vi "practica4rio.vi"() -> ()   [LabVIEW 2017]
uses:
  <vilib>/addons/Fuzzy Logic/FL Fuzzy Controller (SIMO).vi
  <vilib>/addons/Fuzzy Logic/NI_Fuzzy_Logic_API.lvlib
panel:
  out "motor izquierdo":dbl[](graph)
  out "motor derecho":dbl[](graph)
  in  "file path 2":path
  in  "Reset":bool
  out "Distancia":dbl
  out "Angulo":dbl
  out "Motor Izquierda":dbl(slide) scale=-100.0..100.0
  out "Motor Derecha":dbl(slide) scale=-100.0..100.0
  out "Plano de trabajo":picture
  in  "stop":bool
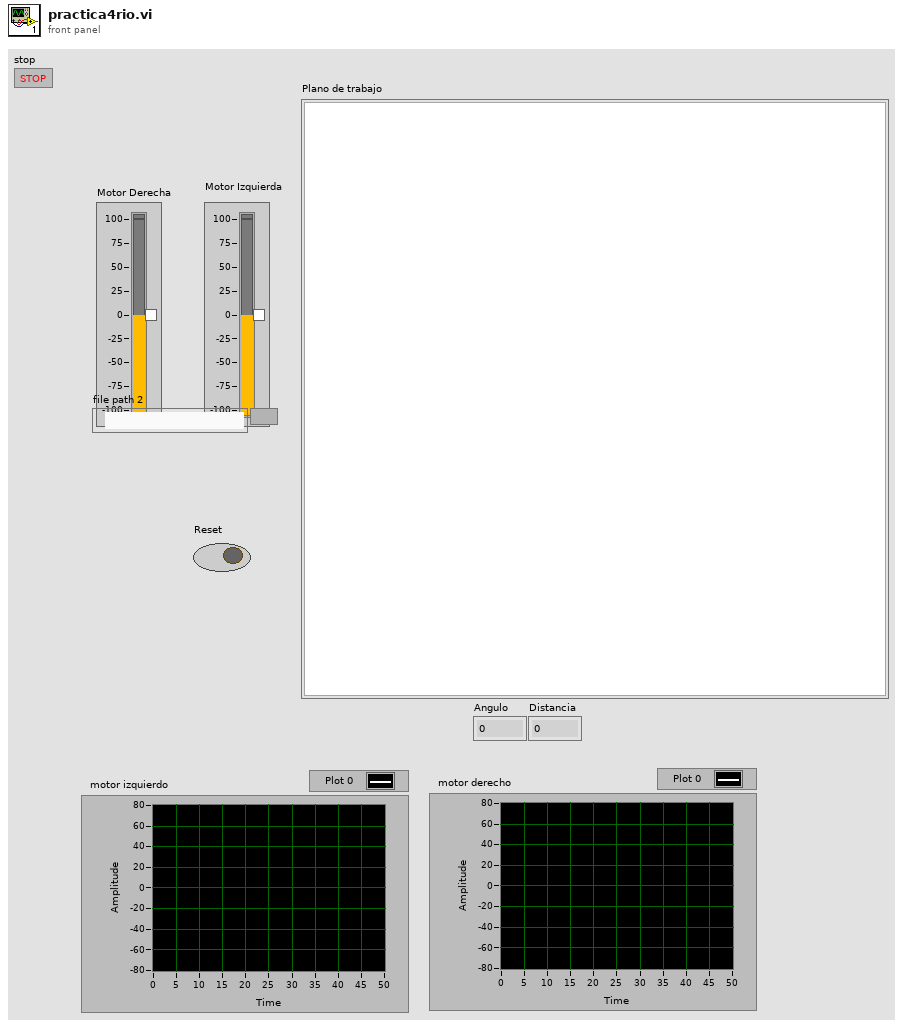
[diagram p1: front panel]
types:
  T1 = typedef "NI_Fuzzy_Logic_API.lvlib/FL System.ctl" = cluster{"input variables":T2[], "output variables":T2[], "rules":T5[], "defuzzification method":T11, "description":string, "user MF interpolating polynomials":T12[]}
  T2 = typedef "NI_Fuzzy_Logic_API.lvlib/FL Variable.ctl" = cluster{"name":string, "range":dbl[], "MFs":T3[]}
  T3 = typedef "NI_Fuzzy_Logic_API.lvlib/FL Membership Function.ctl" = cluster{"name":string, "shape":T4, "points":dbl[], "color":u32, "user-defined shape index":i32}
  T4 = typedef "NI_Fuzzy_Logic_API.lvlib/FL Membership Function Shape.ctl" = u16
  T5 = typedef "NI_Fuzzy_Logic_API.lvlib/FL Rule.ctl" = cluster{"antecedents":T6[], "antecedent connective":T8, "consequents":T9[], "consequent implication":T10, "degree of support":dbl}
  T6 = typedef "NI_Fuzzy_Logic_API.lvlib/FL Antecedent.ctl" = cluster{"Var Index":i32, "MF Index":i32, "Cond":T7}
  T7 = typedef "NI_Fuzzy_Logic_API.lvlib/FL Modifier.ctl" = u16
  T8 = typedef "NI_Fuzzy_Logic_API.lvlib/FL Antecedent Connective.ctl" = u16
  T9 = typedef "NI_Fuzzy_Logic_API.lvlib/FL Consequent.ctl" = cluster{"Var Index":i32, "MF Index":i32, "Cond":T7}
  T10 = typedef "NI_Fuzzy_Logic_API.lvlib/FL Consequent Implication.ctl" = u16
  T11 = typedef "NI_Fuzzy_Logic_API.lvlib/FL Defuzzification.ctl" = u16
  T12 = typedef "NI_Fuzzy_Logic_API.lvlib/FL Interpolating polynomials.ctl" = cluster{"X":dbl[], "Y":dbl[], "Y(x) coeff":dbl[][], "X(y) coeff":dbl[][], "Area(y) coeff":dbl[][], "coa_x(y) coeff":dbl[][]}
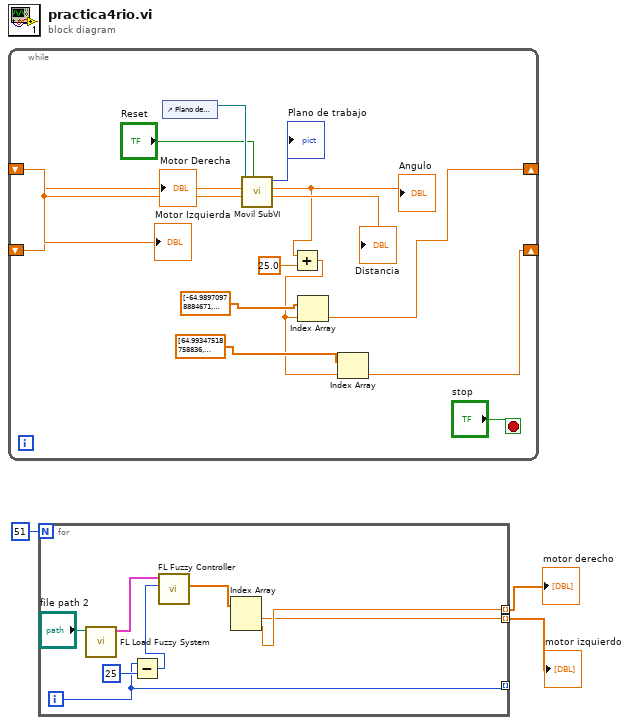
[diagram p0: block diagram]
diagram:
  n1 = while {
    shift-right: [w8] -> _
    shift-left: _ -> [w12]
    shift-right: [w7] -> _
    shift-left: _ -> [w11]
    stop <- "stop" stop-if-true
    n2 = control-ref of="Plano de trabajo"() -> (w15:refnum<vi>)
    n3 = call "Movil SubVI.vi"("Reset"="Reset", "Motor Izquierda"=w12, "Motor Derecha"=w11, "Ref Plano"=w15) -> ("Distancia"=→"Distancia":dbl, "Angulo"=w5:dbl, "Plano de trabajo"=→"Plano de trabajo":picture)  [unwired: 3 in, 2 out]
    "Angulo" <- w5
    n4 = Add(x=w5, y=25.0) -> (x+y=w4:dbl)
    n5 = Index Array(array=dbl[] [-64.98970978884671, -64.98970978884671, -64.98970978884671, -64.98970978884671, -64.98970978884671, -64.98970978884671, -64.98970978884671, -64.98970978884671, -64.98970978884671, -64.98970978884671, -64.98970978884671, -64.35040426567848, -63.631690929812855, -62.84813012868776, -61.99715300975148, -61.102841729064856, -60.15367255138196, -59.15251596821936, -58.12132266011543, -57.03161255798153, -55.947901216976796, -49.159265034917624, -40.68105539314433, -32.87765939556559, -21.145718077893275, -0.2111189303307497, 20.81360607853993, 32.35119819252564, 40.163689835295, 48.75489419549819, 55.937920853620646, 57.04886048496055, 58.0999370638831, 59.15888049075932, 60.151030157285845, 61.09835496004473, 62.00022165797324, 62.84478898617338, 63.631531974855626, 64.346991084973, 64.99347518758836, 64.99347518758836, 64.99347518758836, 64.99347518758836, 64.99347518758836, 64.99347518758836, 64.99347518758836, 64.99347518758836, 64.99347518758836, 64.99347518758836, 64.99347518758836] ("Waveform Graph 4"), index=w4) -> (element=w8:dbl)
    n6 = Index Array(array=dbl[] [64.99347518758836, 64.99347518758836, 64.99347518758836, 64.99347518758836, 64.99347518758836, 64.99347518758836, 64.99347518758836, 64.99347518758836, 64.99347518758836, 64.99347518758836, 64.99347518758836, 64.346991084973, 63.631531974855626, 62.84478898617338, 62.00022165797324, 61.09835496004473, 60.151030157285845, 59.15888049075932, 58.0999370638831, 57.04886048496055, 55.937920853620646, 48.75489419549819, 40.163689835295, 32.35119819252564, 20.81360607853993, -0.2111189303307497, -21.145718077893275, -32.87765939556559, -40.68105539314433, -49.159265034917624, -55.947901216976796, -57.03161255798153, -58.12132266011543, -59.15251596821936, -60.15367255138196, -61.102841729064856, -61.99715300975148, -62.84813012868776, -63.631690929812855, -64.35040426567848, -64.98970978884671, -64.98970978884671, -64.98970978884671, -64.98970978884671, -64.98970978884671, -64.98970978884671, -64.98970978884671, -64.98970978884671, -64.98970978884671, -64.98970978884671, -64.98970978884671] ("Waveform Graph 3"), index=w4) -> (element=w7:dbl)
    "Motor Derecha" <- w11
    "Motor Izquierda" <- w12
  }
  n7 = for {
    N: 51 -> [_]
    tunnel: [w22] -> w1 mode=indexing
    tunnel: [w21] -> w2 mode=indexing
    tunnel: [w18] -> _ mode=indexing
    i -> [w18]
    n8 = call <vilib>:"FL Load Fuzzy System.vi"("file path"="file path 2") -> ("fuzzy system out"=w24:T1)  [unwired: 9 in, 1 out]
    n9 = Subtract(x=w18, y=25) -> (x-y=w19:i32)
    n10 = call-poly <vilib>:"FL Fuzzy Controller.vi"("input value"=w19, "fuzzy system in"=w24) -> ("output values"=w23:dbl[])  [unwired: 5 in, 4 out]
    n11 = Index Array(array=w23) -> (element #1=w21:dbl, element #2=w22:dbl)  [unwired: 2 in]
  }
  "motor derecho" <- w1
  "motor izquierdo" <- w2
